vi "Open.vi"(8 "error in (no error)":errorcluster, 9 "Markdown Images Dir":path, 10 "Markdown (*.md)":path, 11 "Library (*.lvlib)":path) -> (0 "error out":errorcluster)   [LabVIEW 2018, in "Markdown.lvlib"]
doc: "Initialize the markdown generator, resets the global variables and resolves the markdown paths.\n\nUse `%name%` to replace the Library name (without extension) in the output filepaths."
uses:
  Markdown.lvlib
  Global.vi
  TypeDefs/Item.ctl
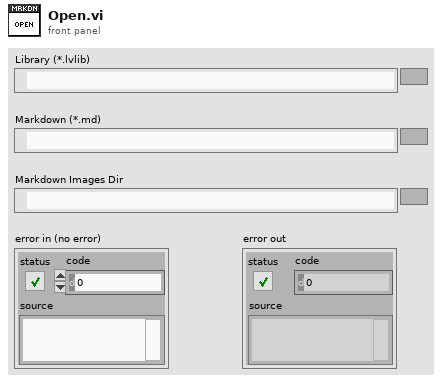
[diagram p1: front panel]
types:
  T1 = typedef "Markdown.lvlib/Item.ctl" = cluster{"Name":string, "Icon":picture, "Path":path, "Title":string, "Desc":string, "ConPane":picture, "TypeString":string, "ProjectItem":string, "VI Type":enum32{"invalid VI type", "Standard VI", "Control VI", "Global VI", "Polymorphic VI", "Configuration VI", "SubSystem", "Facade VI", "Method VI", "Statechart Diagram VI"}}
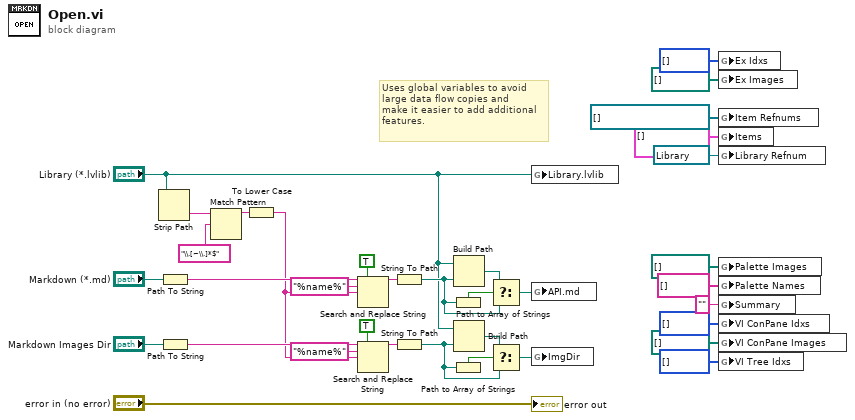
[diagram p0: block diagram]
diagram:
  # "Uses global variables to avoid\nlarge data flow copies and\nmake it easier to add additional\nfeatures."
  n1 = Strip Path(path="Library (*.lvlib)") -> (name=w3:string)  [unwired: 1 out]
  n2 = Path To String(path="Markdown (*.md)") -> (string=w15:string)
  n3 = Path To String(path="Markdown Images Dir") -> (string=w7:string)
  n4 = Match Pattern(string=w3, regular expression="\\.[~\\.]*$") -> (before substring=w1:string)  [unwired: 4 out]
  n5 = To Lower Case(string=w1) -> (all lower case string=w4:string)
  n6 = Search and Replace String(replace all?=TRUE ("replace all? (F)"), input string=w15, search string="%name%", replace string=w4) -> (result string=w12:string)  [unwired: 4 in, 3 out]
  n7 = Search and Replace String(replace all?=TRUE ("replace all? (F)"), input string=w7, search string="%name%", replace string=w4) -> (result string=w6:string)  [unwired: 4 in, 3 out]
  n8 = String To Path(string=w12) -> (path=w13:path)
  n9 = String To Path(string=w6) -> (path=w14:path)
  n10 = Path to Array of Strings(0:w13) -> (1:w34:bool)  [unwired: 1 out]
  n11 = Path to Array of Strings(0:w14) -> (1:w31:bool)  [unwired: 1 out]
  n12 = Build Path(base path="Library (*.lvlib)", name or relative path=w13) -> (appended path=w33:path)
  n13 = Build Path(base path="Library (*.lvlib)", name or relative path=w14) -> (appended path=w32:path)
  n14 = Select(t=w33, s=w34, f=w13) -> (s? t:f=w28:path)
  n15 = Select(t=w32, s=w31, f=w14) -> (s? t:f=w25:path)
  n16 = global write "Global.vi" "Library.lvlib"("Library (*.lvlib)") -> ()
  n17 = global write "Global.vi" "API.md"(w28) -> ()
  n18 = global write "Global.vi" "ImgDir"(w25) -> ()
  n19 = global write "Global.vi" "Ex Idxs"(i32[] [] ("Ex Idxs")) -> ()
  n20 = global write "Global.vi" "Ex Images"(path[] [] ("Ex Images")) -> ()
  n21 = global write "Global.vi" "Item Refnums"(refnum<vi>[] [] ("Item Refnums")) -> ()
  n22 = global write "Global.vi" "Items"(T1[] [] ("Items")) -> ()
  n23 = global write "Global.vi" "Library Refnum"(refnum<vi> refnum ("Library Refnum")) -> ()
  n24 = global write "Global.vi" "Palette Images"(path[] [] ("Palette Images")) -> ()
  n25 = global write "Global.vi" "Palette Names"(string[] [] ("Palette Names")) -> ()
  n26 = global write "Global.vi" "Summary"("" ("Summary")) -> ()
  n27 = global write "Global.vi" "VI ConPane Idxs"(i32[] [] ("VI ConPane Idxs")) -> ()
  n28 = global write "Global.vi" "VI ConPane Images"(path[] [] ("VI ConPane Images")) -> ()
  n29 = global write "Global.vi" "VI Tree Idxs"(i32[] [] ("VI Tree Idxs")) -> ()
  "error out" <- "error in (no error)"
